vi "Disconnect.vi"(8 "error in":errorcluster, 11 "MiniIO in":refnum<class "MiniIO.lvclass">) -> (0 "error out":errorcluster, 3 "MiniIO out":refnum<class "MiniIO.lvclass">)   [LabVIEW 2018, in "MiniIO.lvlib" / "MiniIO.lvclass"]
uses:
  MiniIO.lvclass
  MiniIO.lvclass/MiniIO.ctl
  <vilib>/NI/Modbus Library/API/Master/Modbus Master.lvclass
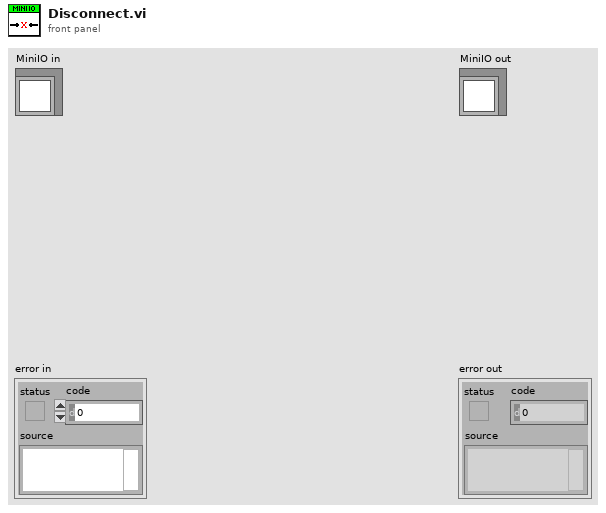
[diagram p1: front panel]
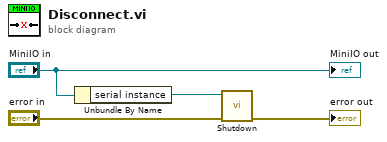
[diagram p0: block diagram]
diagram:
  n1 = Unbundle By Name("MiniIO in") -> ("serial instance"=w3:refnum<class "Modbus Master.lvclass">)
  n2 = call-dynamic "Shutdown.vi"("error in"="error in", "Modbus master in"=w3) -> ("error out"=→"error out":errorcluster)  [unwired: 9 in]
  "MiniIO out" <- "MiniIO in"
